vi "MecanumCalculate.vi"(9 "Rotate":dbl, 10 "Strafe":dbl, 11 "Forward":dbl) -> (0 "BackRight":dbl, 1 "BackLeft":dbl, 2 "FrontRight":dbl, 3 "FrontLeft":dbl)   [LabVIEW 2012]
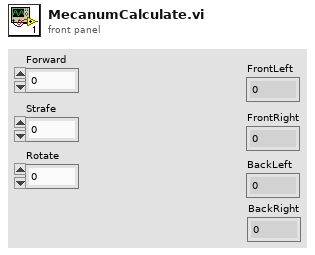
[diagram p1: front panel]
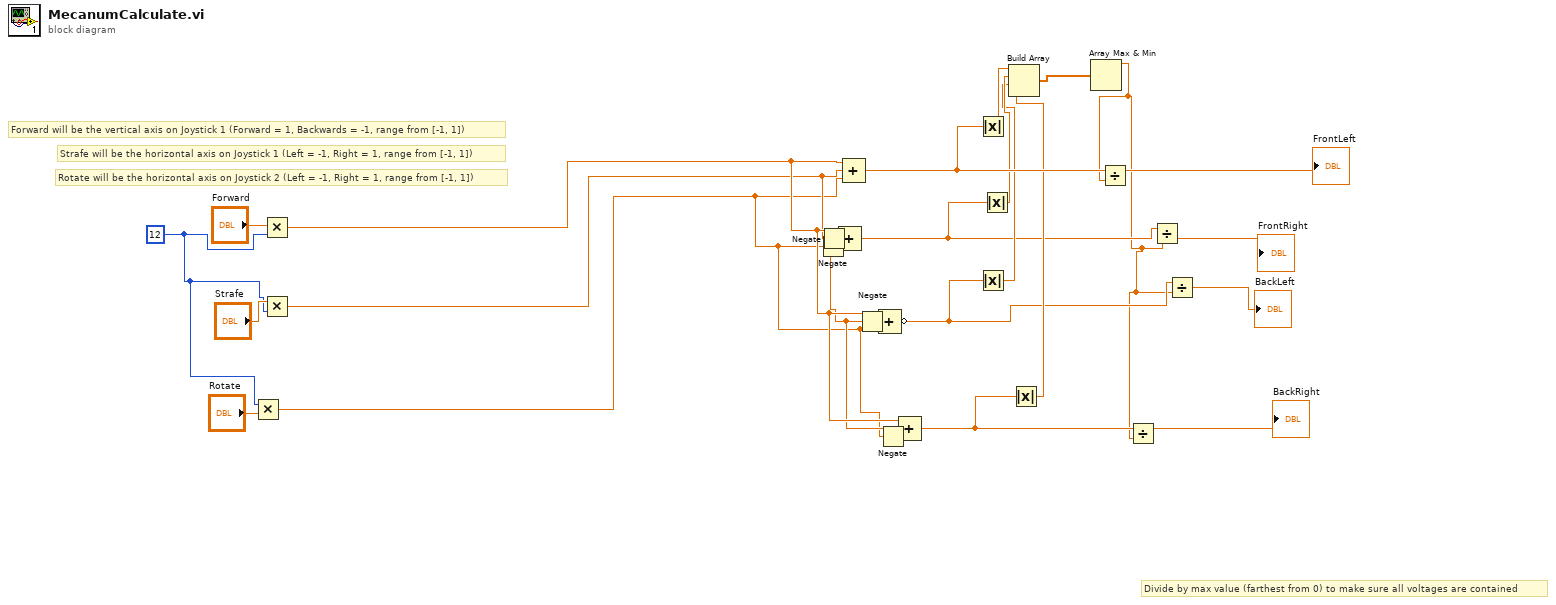
[diagram p0: block diagram]
diagram:
  w22 = 12
  # "Divide by max value (farthest from 0) to make sure all voltages are contained"
  # "Rotate will be the horizontal axis on Joystick 2 (Left = -1, Right = 1, range from [-1, 1])"
  # "Strafe will be the horizontal axis on Joystick 1 (Left = -1, Right = 1, range from [-1, 1])"
  # "Forward will be the vertical axis on Joystick 1 (Forward = 1, Backwards = -1, range from [-1, 1])"
  n1 = Multiply(x=w22, y="Rotate") -> (x*y=w19:dbl)
  n2 = Multiply(x="Forward", y=w22) -> (x*y=w21:dbl)
  n3 = Multiply(x="Strafe", y=w22) -> (x*y=w20:dbl)
  n4 = Negate(x=w19) -> (-x=w17:dbl)
  n5 = Negate(x=w20) -> (-x=w18:dbl)
  n6 = Compound Arithmetic op=ADD(w21, w18, w17) -> (w5:dbl)
  n7 = Compound Arithmetic op=ADD(w21, w20, w19) -> (w14:dbl)
  n8 = Negate(x=w20) -> (-x=w16:dbl)
  n9 = Negate(x=w19) -> (-x=w15:dbl)
  n10 = Compound Arithmetic op=ADD(w21, w16, w19) -> (invert w4:dbl)
  n11 = Compound Arithmetic op=ADD(w21, w20, w15) -> (w13:dbl)
  n12 = Absolute Value(x=w14) -> (abs(x)=w12:dbl)
  n13 = Absolute Value(x=w4) -> (abs(x)=w10:dbl)
  n14 = Absolute Value(x=w5) -> (abs(x)=w11:dbl)
  n15 = Absolute Value(x=w13) -> (abs(x)=w9:dbl)
  n16 = Build Array(w12, w11, w10, w9) -> (w8:dbl[])
  n17 = Array Max & Min(array=w8) -> (max value=w1:dbl)  [unwired: 3 out]
  n18 = Divide(x=w14, y=w1) -> (x/y=→"FrontLeft":dbl)
  n19 = Divide(x=w13, y=w1) -> (x/y=→"BackRight":dbl)
  n20 = Divide(x=w5, y=w1) -> (x/y=→"FrontRight":dbl)
  n21 = Divide(x=w4, y=w1) -> (x/y=→"BackLeft":dbl)
